vi "INI Build Ring Text Information.vi"(0 "Type Descriptor":i16[](array[numeric])=[126, 16406, 15, 2125, 24952, 8259, 26721, 29188, 22121, 25975, 845, 26990, 845, 24952, 1108, 31088, 25860, 21605, 30836, 1106, 28527, 29699, 17513, 29193, 21605, 30836, 8268, 26995, 29700, 20594, 25955, 2628, 26989, 25966, 29545, 28526, 29449, 17513, 27936, 21353, 31333, 29450, 17513, 27936, 19553, 25189, 27763, 2889, 29797, 27936, 19553, 25189, 27763, 2386, 25971, 27002, 24930, 27749, 2384, 24946, 29541, 8276, 24935] format="%.0x", 11 "Error In (no error)":errorcluster) -> (4 "Ring Text":string, 6 "Ring Text Items":string[](array[string]), 15 "Error Out":errorcluster)   [LabVIEW 2011]
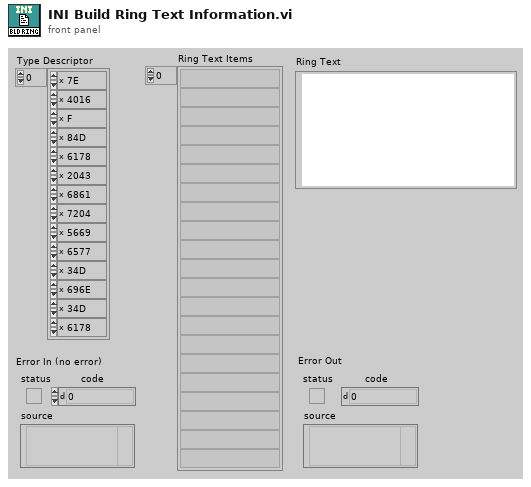
[diagram p1: front panel]
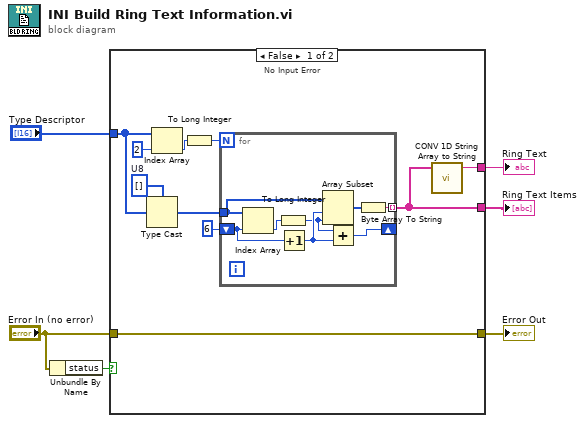
[diagram p0: block diagram]
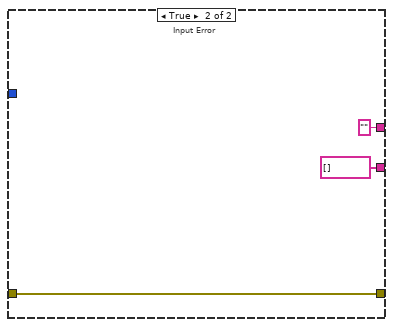
[diagram p2: hidden frame]
diagram:
  n1 = Unbundle By Name("Error In (no error)") -> ("status"=w6:bool)
  n2 = case shown="False" w6 {
    tunnel: [w16 w27] -> w5
    tunnel: "Error In (no error)" -> [w16 w27]
    tunnel: "Type Descriptor" -> [w12 _]
    tunnel: [w8 string[] []] -> w2
    tunnel: [w7 "" ("String")] -> w1
    frame False {
      w10 = u8[] []  # U8
      # "No Input Error"
      n3 = Type Cast(type=w10, x=w12) -> (*(type *) &x=w11:u8[])
      n4 = Index Array(array=w12, index=2 ("Index")) -> (element=w14:i16)
      n5 = To Long Integer(number=w14) -> (32bit integer=w13:i32)
      n6 = for {
        N: w13 -> [_]
        tunnel: w11 -> [w24]
        shift-right: [w19] -> _
        shift-left: 6 ("Index") -> [w22]
        tunnel: [w17] -> w8 mode=indexing
        n7 = Index Array(array=w24, index=w22) -> (element=w23:u8)
        n8 = To Long Integer(number=w23) -> (32bit integer=w20:i32)
        n9 = Increment(x=w22) -> (x+1=w21:i32)
        n10 = Array Subset(array=w24, index=w21, length=w20) -> (w18:u8[])
        n11 = Add(x=w20, y=w21) -> (x+y=w19:i32)
        n12 = Byte Array To String(unsigned byte array=w18) -> (string=w17:string)
      }
      n13 = call "CONV 1D String Array to String.vi"("1-D String"=w8) -> ("String"=w7:string)  [unwired: 1 in, 7 out]
    }
    frame True {
      # "Input Error"
    }
  }
  "Error Out" <- w5
  "Ring Text" <- w1
  "Ring Text Items" <- w2
